vi "format error for pallet sent to repair from glass set station.vi"(11 "iGPS overall results":T1) -> (3 "Error Data":string[](array[string]))   [LabVIEW 2018]
uses:
  02.Type Def's/iGPS overall results.ctl
  02.Type Def's/iGPS channel result.ctl
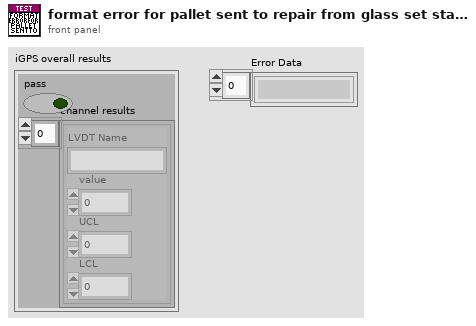
[diagram p1: front panel]
types:
  T1 = typedef "iGPS overall results.ctl" = cluster{"pass":bool, "channel results":T2[]}
  T2 = typedef "iGPS channel result.ctl" = cluster{"LVDT Name":string, "value":sgl, "UCL":sgl, "LCL":sgl}
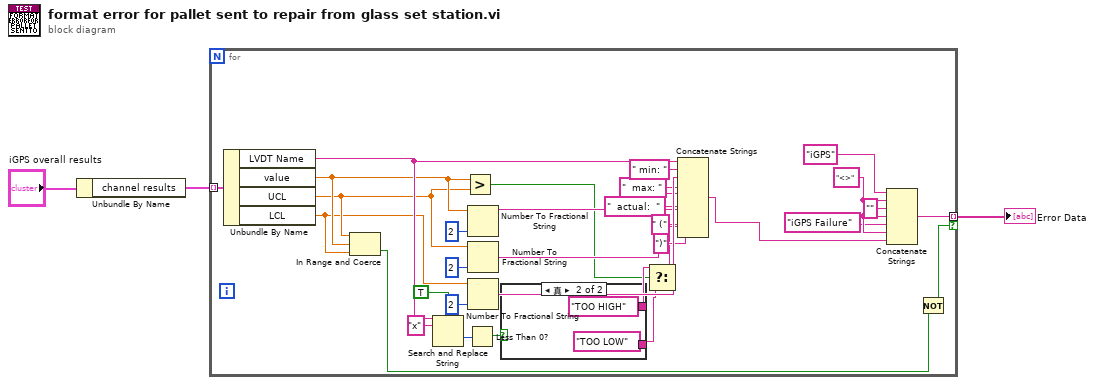
[diagram p0: block diagram]
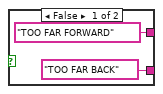
[diagram p2: hidden frame]
diagram:
  n1 = Unbundle By Name("iGPS overall results") -> ("channel results"=w3:T2[])
  n2 = for {
    tunnel: w3 -> [w35] mode=indexing
    tunnel: [w9] -> w1 mode=indexing if=w7
    w30 = "<>"
    n3 = Unbundle By Name(w35) -> ("LVDT Name"=w34:string, "value"=w33:sgl, "UCL"=w32:sgl, "LCL"=w31:sgl)
    n4 = In Range and Coerce(upper limit=w32, x=w33, lower limit=w31) -> (In Range?=w8:bool)  [unwired: 1 out]
    n5 = Search and Replace String(case sensitive?=TRUE ("ignore case? (F)"), input string=w34, search string="x") -> (offset past replacement=w12:i32)  [unwired: 5 in, 3 out]
    n6 = Greater?(x=w33, y=w32) -> (0:w14:bool)
    n7 = Less Than 0?(x=w12) -> (x < 0?=w11:bool)
    n8 = Number To Fractional String(number=w33, precision (6)=i16 2) -> (F-format string=w20:string)  [unwired: 2 in]
    n9 = Number To Fractional String(number=w32, precision (6)=i16 2) -> (F-format string=w22:string)  [unwired: 2 in]
    n10 = Number To Fractional String(number=w31, precision (6)=i16 2) -> (F-format string=w24:string)  [unwired: 2 in]
    n11 = case shown="真" w11 {
      tunnel: ["TOO FAR FORWARD" ("string") "TOO HIGH" ("string")] -> w16
      tunnel: ["TOO FAR BACK" ("string") "TOO LOW" ("string")] -> w15
      frame False {
      }
      frame True {
      }
    }
    n12 = Select(t=w16, s=w14, f=w15) -> (s? t:f=w17:string)
    n13 = Concatenate Strings(w34, " min: " ("string"), w24, "  max: " ("string"), w22, "  actual:  " ("string"), w20, " (" ("string"), w17, ")" ("string")) -> (w5:string)
    n14 = Concatenate Strings("iGPS", w30, "" ("string"), w30, "iGPS Failure", w30, w5) -> (w9:string)
    n15 = Not(x=w8) -> (.not. x?=w7:bool)
  }
  "Error Data" <- w1
